vi "Fill From Traces.vi"(8 "Error In":errorcluster, 9 "Settings":T1[](array[typedef]), 11 "Tree Control In":refnum<vi>) -> (0 "Error Out":errorcluster, 3 "Tree Control Out":refnum<vi>)   [LabVIEW 2018, in "TraceTreeEditor.lvlib"]
uses:
  TraceTreeEditor.lvlib
  TracerLibrary/Tracer/TraceItemDefinition.ctl
  TracerLibrary/Tracer/Tracer.lvclass
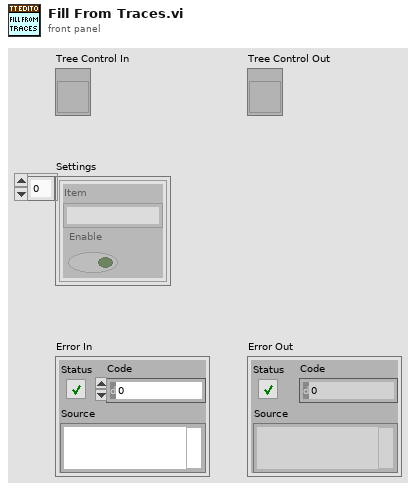
[diagram p1: front panel]
types:
  T1 = typedef "TracerLibrary.lvlib/Tracer.lvclass/TraceItemDefinition.ctl" = cluster{"Item":string, "Enable":bool}
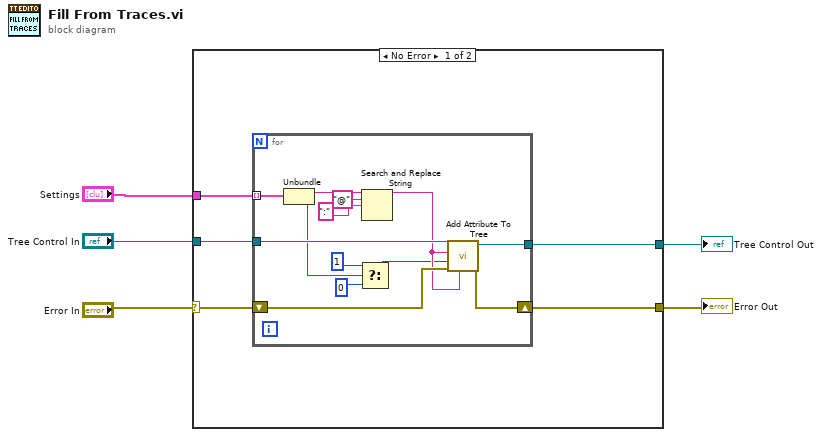
[diagram p0: block diagram]
diagram:
  n1 = case shown="No Error" "Error In" {
    selector: "Error In" -> [w10 w24]
    tunnel: [w8 _] -> w3
    tunnel: "Tree Control In" -> [w7 _]
    tunnel: "Settings" -> [w6 _]
    tunnel: [w9 w24] -> w4
    frame No Error {
      n2 = for {
        tunnel: w7 -> [w21]
        tunnel: w6 -> [w20] mode=indexing
        tunnel: [w11] -> w8
        shift-right: [w22] -> w9
        shift-left: w10 -> [w23]
        n3 = Unbundle(w20) -> ("Item"=w19:string, "Enable"=w13:bool)
        n4 = Select(t=1 ("y"), s=w13, f=0 ("y")) -> (s? t:f=w12:i32)
        n5 = Search and Replace String(input string=w19, search string="@", replace string=":" ("search string")) -> (result string=w16:string)  [unwired: 5 in, 3 out]
        n6 = call "Add Attribute To Tree.vi"("Display Name"=w16, "Error In"=w23, "Active Item:Symbol Index"=w12, "Attribute Name"=w16, "Attribute Table In"=w21) -> ("Error Out"=w22:errorcluster, "Attribute Table Out"=w11:refnum<vi>)  [unwired: 5 in]
      }
    }
    frame Error {
    }
  }
  "Tree Control Out" <- w3
  "Error Out" <- w4
